vi "Exemple_Metrics_Precision_Recall_Curve.vi"() -> ()   [LabVIEW 2020]
uses:
  Objet/3 - Model selection and evaluation/3.3 - Metrics and scoring/precision_recall_curve/Precision_Recall_Curve.vi
panel:
  out "Data":T1
  out "error out":errorcluster caption="sortie d'erreur"
  in  "error in (no error)":errorcluster caption="entrée d'erreur (pas d'erreur)"
  in  "precision_recall_curve":T2={"pos_label"={"dtype_pos_label"="None", "pos_label"="None"}, "sample_weight"=[], "Returns"="precision"}
  in  "probas_pred":string[][](array[string])=[["0,1"], ["0,4"], ["0,35"], ["0,8"]]
  in  "y_true":string[][](array[string])=[["0"], ["0"], ["1"], ["1"]]
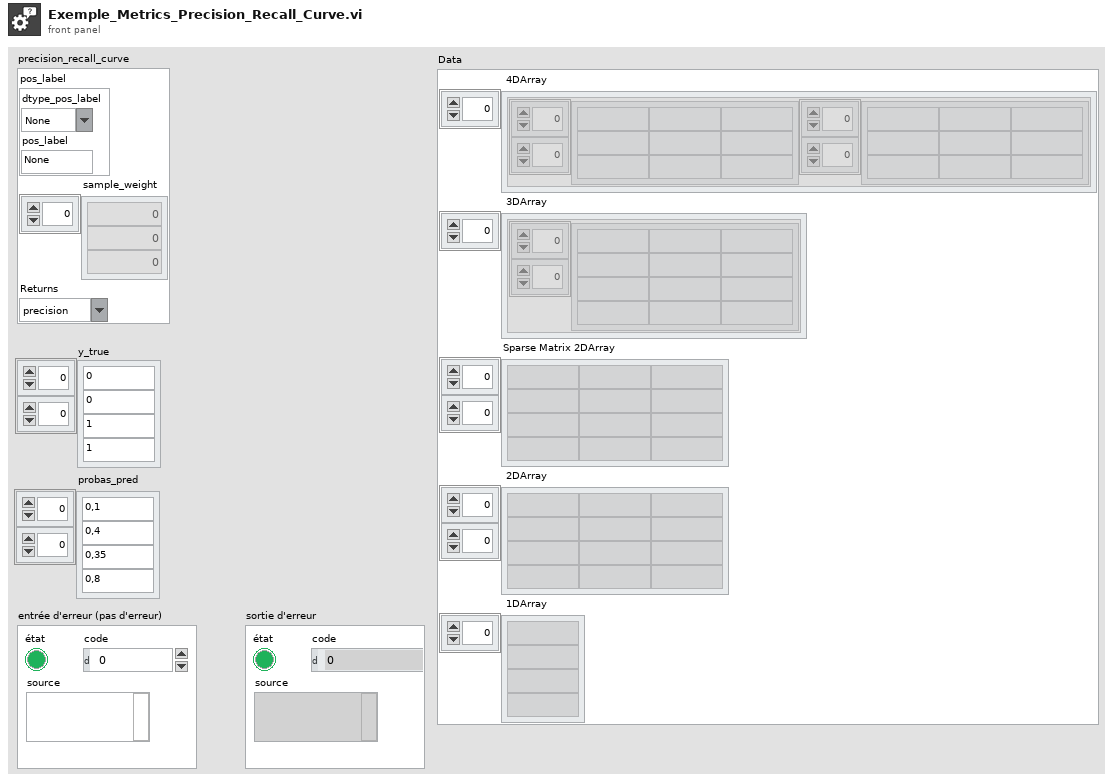
[diagram p1: front panel]
types:
  T1 = cluster{" 4DArray":cluster{"1":string[][], "2":string[][]}[], " 3DArray":cluster{"Tableau":string[][]}[], "Sparse Matrix 2DArray":string[][], " 2DArray":string[][], " 1DArray":string[]}
  T2 = cluster{"pos_label":cluster{"dtype_pos_label":string, "pos_label":string}, "sample_weight":dbl[], "Returns":string}
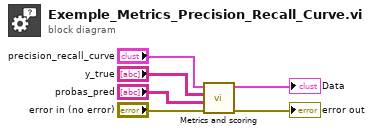
[diagram p0: block diagram]
diagram:
  n1 = call-poly "Metrics and scoring.vi"("error in (no error)"="error in (no error)", "probas_pred"="probas_pred", "y_true"="y_true", "precision_recall_curve"="precision_recall_curve") -> ("error out"=→"error out":errorcluster, "Data"=→"Data":T1)  [unwired: 6 in]
